vi "CheckForSec.vi"(6 "Scan Info":T1 {"delay" format="%.2f"; "pivot distance" format="%.2f"; "sector scan angle" format="%.2f"}, 8 "Last sector file opened":path, 9 "Current file":path) -> (2 "sector?":bool, 3 "= 360?":bool)   [LabVIEW 2022 SP3]
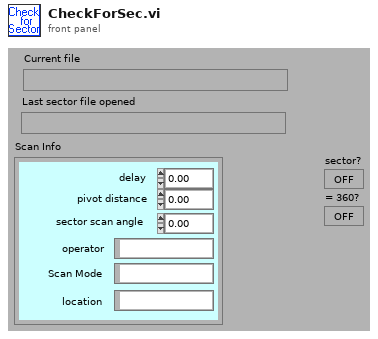
[diagram p1: front panel]
types:
  T1 = cluster{"delay":sgl, "pivot distance":sgl, "sector scan angle":sgl, "operator":string, "Scan Mode":string, "location":string}
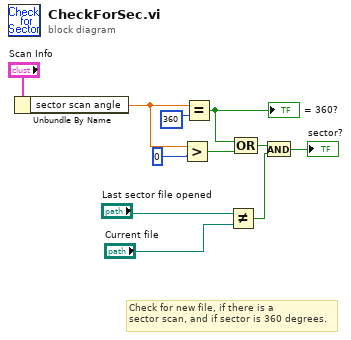
[diagram p0: block diagram]
diagram:
  # "Check for new file, if there is a\nsector scan, and if sector is 360 degrees."
  n1 = Unbundle By Name("Scan Info") -> ("sector scan angle"=w5:sgl)
  n2 = Greater?(x=w5, y=0) -> (0:w2:bool)
  n3 = Equal?(x=w5, y=360) -> (x = y?=w3:bool)
  "= 360?" <- w3
  n4 = Not Equal?(x="Last sector file opened", y="Current file") -> (x != y?=w9:bool)
  n5 = Compound Arithmetic op=OR(w3, w2) -> (w1:bool)
  n6 = And(x=w1, y=w9) -> (x .and. y?=→"sector?":bool)
